vi "Close_Instr.vi"(8 "error in (no error)":errorcluster caption="entrée d'erreur (pas d'erreur)", 11 "Class Instrument Firebase en entrée":refnum<class "Class Instrument Database Altyor.lvclass">) -> (0 "error out":errorcluster caption="sortie d'erreur", 3 "Class Instrument Firebase en sortie":refnum<class "Class Instrument Database Altyor.lvclass">)   [LabVIEW 2020, in "Library Instrument & Equipement.lvlib" / "Library Instruments.lvlib" / "Class Instrument Database Altyor.lvclass"]
uses:
  Class Instrument Database Altyor.lvclass
  Class Instrument Database Altyor.lvclass/Class Instrument Database Altyor.ctl
  Database/Database Altyor/Database Altyor.lvclass
  Instrument (Default)/Class Instrument (Default).lvclass
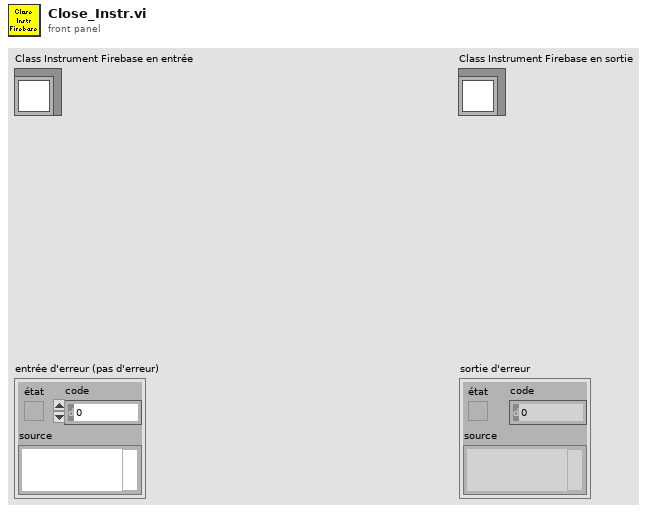
[diagram p1: front panel]
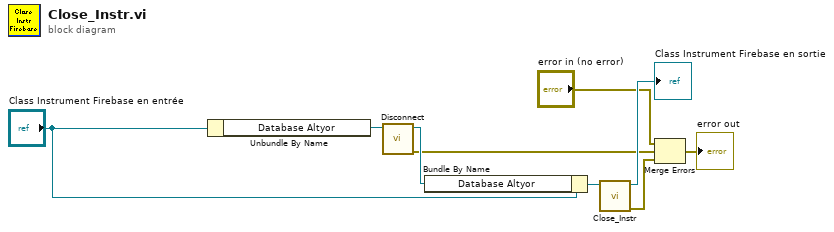
[diagram p0: block diagram]
diagram:
  n1 = Unbundle By Name("Class Instrument Firebase en entrée") -> ("Database Altyor"=w3:refnum<class "Database Altyor.lvclass">)
  n2 = call-dynamic "Disconnect.vi"("Database Altyor en entrée"=w3) -> ("error out"=w1:errorcluster, "Database Altyor en sortie"=w2:refnum<class "Database Altyor.lvclass">)  [unwired: 9 in]
  n3 = Bundle By Name(cluster="Class Instrument Firebase en entrée", "Database Altyor"=w2) -> (w7:refnum<class "Class Instrument Database Altyor.lvclass">)
  n4 = call-parent "Close_Instr.vi"("Class Instrument (Default) en entrée"=w7) -> ("error out"=w6:errorcluster, "Class Instrument (Default) en sortie"=→"Class Instrument Firebase en sortie":refnum<class "Class Instrument Database Altyor.lvclass">)  [unwired: 9 in]
  n5 = Merge Errors("error in (no error)", w1, w6) -> (→"error out":errorcluster)
